vi "getReturnCodes.vi"(8 "error in (no error)":errorcluster, 11 "SUBACK in":refnum<class "SUBACK.lvclass">) -> (0 "error out":errorcluster, 2 "Subscription Success":T1[](array[typedef]), 3 "SUBACK out":refnum<class "SUBACK.lvclass">)   [LabVIEW 2013, in "MQTT_Control_Packets.lvlib" / "SUBACK.lvclass"]
uses:
  SUBACK.lvclass
  Subscription Success Code.ctl
  ControlPacket/QualityOfService -- enum.ctl
  ControlPacket/ControlPacket.lvclass/ControlPacket.ctl
  ControlPacket/ControlPacket.lvclass
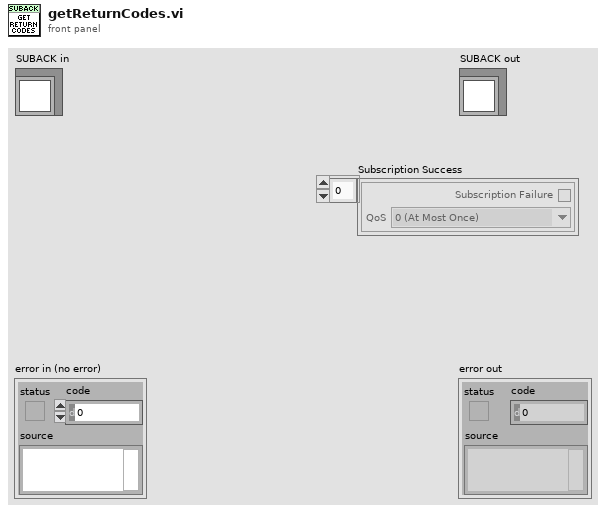
[diagram p1: front panel]
types:
  T1 = typedef "MQTT_Control_Packets.lvlib/SUBACK.lvclass/Subscription Success Code.ctl" = cluster{"Subscription Failure":bool, "QoS":T2}
  T2 = typedef "MQTT_Control_Packets.lvlib/ControlPacket.lvclass/QualityOfService -- enum.ctl" = enum16{"0 (At Most Once)", "1 (At Least Once)", "2 (Exactly Once)"}
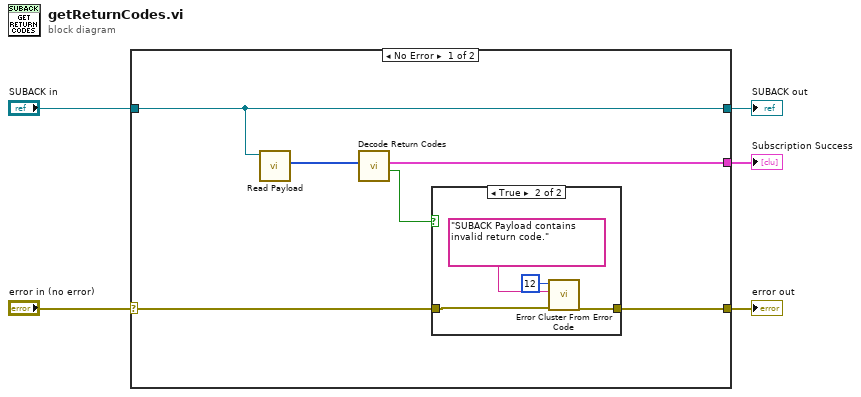
[diagram p0: block diagram]
diagram:
  n1 = case shown="No Error" "error in (no error)" {
    selector: "error in (no error)" -> [w8 w18]
    tunnel: [w7 w18] -> w4
    tunnel: [w11 w17] -> w2
    tunnel: "SUBACK in" -> [w11 w17]
    tunnel: [w9 _] -> w1
    frame No Error {
      n2 = call "Read Payload.vi"("ControlPacket in"=w11) -> ("Payload"=w10:u8[])  [unwired: 9 in, 1 out]
      n3 = call "Decode Return Codes.vi"("Return Codes"=w10) -> ("Invalid Code?"=w6:bool, "Subscription Success"=w9:T1[])  [unwired: 9 in]
      n4 = case shown="True" w6 {
        tunnel: w8 -> [w12 w15]
        tunnel: [w12 w16] -> w7
        frame False {
        }
        frame True {
          n5 = call <vilib>:"Error Cluster From Error Code.vi"("error in (no error)"=w15, "error message (\"\")"="SUBACK Payload contains invalid return code.", "error code (0)"=12) -> ("error out"=w16:errorcluster)  [unwired: 6 in]
        }
      }
    }
    frame Error {
    }
  }
  "error out" <- w4
  "SUBACK out" <- w2
  "Subscription Success" <- w1
